vi "TWM Client Cmd Set Measurement.vi"(7 "end of packet key":string="TWM:command:EndOfPacket", 8 "error in":errorcluster, 9 "processing":T1, 10 "meas":T2, 11 "handle":i32) -> (0 "error out":errorcluster, 3 "handle out":i32)   [LabVIEW 2013, in "TWM Client.lvlib"]
doc: "Write Set measurement command packet to TWM server. Sets measurement configuration and processing configuration. The item \"valid?\" of the cluster(s) must be set to \"True\" to send the setup."
uses:
  TWM Client.lvlib
  TWM Client Meas Setup.ctl
  TWM Client Processing Setup.ctl
  octave/infolib.lvlibp/Private/Add key polymorph parts/EXT.vi
  octave/infolib.lvlibp/Private/Add key polymorph parts/I64.vi
  octave/infolib.lvlibp/Private/Add matrix polymorph parts/1D EXT.vi
  octave/infolib.lvlibp/Private/Add key polymorph parts/String.vi
  octave/infolib.lvlibp/Private/Add matrix polymorph parts/1D String.vi
  octave/infolib.lvlibp
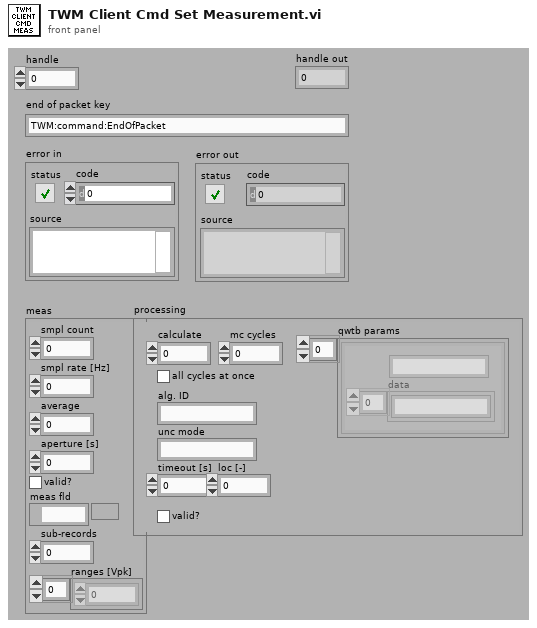
[diagram p1: front panel]
types:
  T1 = typedef "TWM Client.lvlib/TWM Client Processing Setup.ctl" = cluster{"calculate":i32, "all cycles at once":bool, "alg. ID":string, "unc mode":string, "mc cycles":i32, "timeout [s]":dbl, "loc [-]":dbl, "valid?":bool, "qwtb params":cluster{"name":string, "data":string[]}[]}
  T2 = typedef "TWM Client.lvlib/TWM Client Meas Setup.ctl" = cluster{"smpl count":i32, "smpl rate [Hz]":dbl, "average":i32, "aperture [s]":dbl, "valid?":bool, "meas fld":path, "sub-records":i32, "ranges [Vpk]":dbl[]}
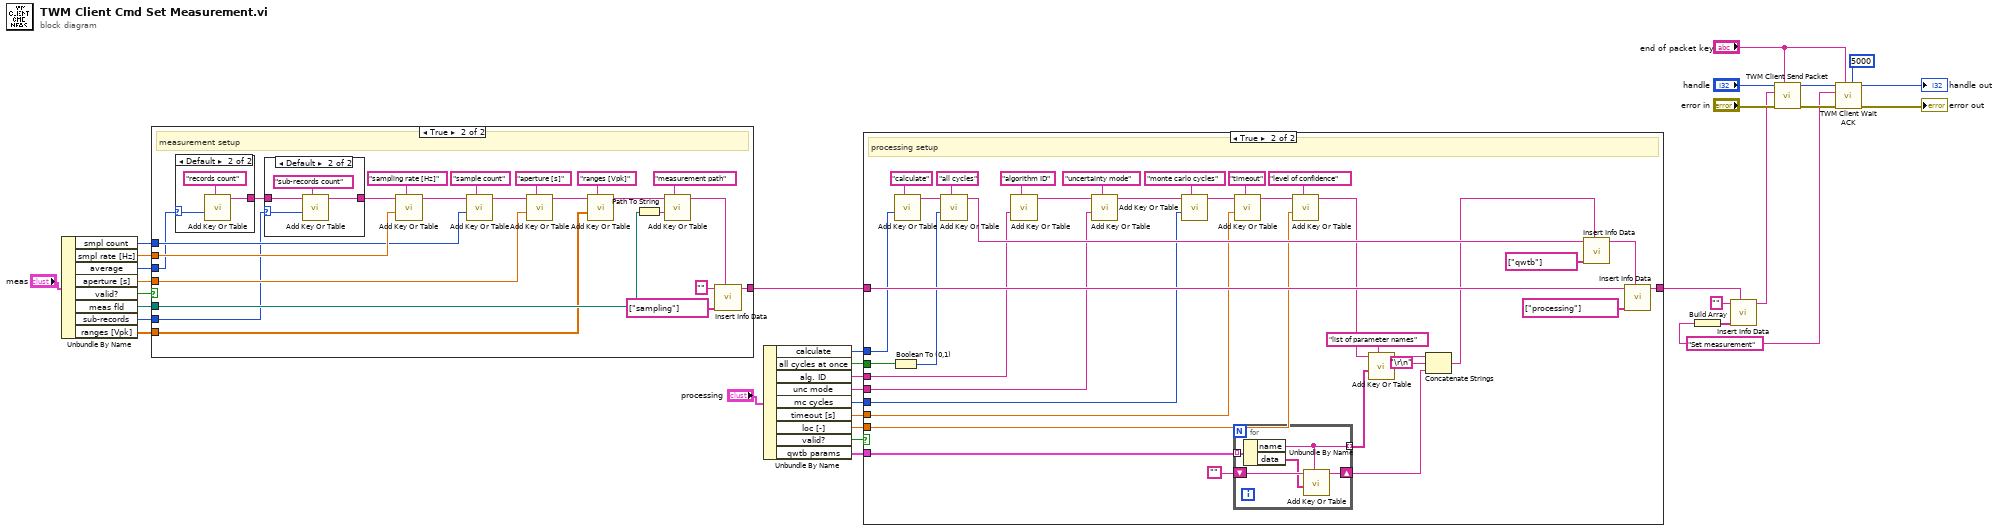
[diagram p0: block diagram]
diagram:
  w3 = "Set measurement" ("section name")
  n1 = Unbundle By Name("meas") -> ("smpl count"=w27:i32, "smpl rate [Hz]"=w28:dbl, "average"=w29:i32, "aperture [s]"=w26:dbl, "valid?"=w25:bool, "meas fld"=w10:path, "sub-records"=w2:i32, "ranges [Vpk]"=w1:dbl[])
  n2 = case shown="True" w25 {
    tunnel: [_ w56] -> w31
    tunnel: w29 -> [_ w39]
    tunnel: w28 -> [_ w51]
    tunnel: w27 -> [_ w50]
    tunnel: w26 -> [_ w49]
    tunnel: w10 -> [_ w44]
    tunnel: w2 -> [_ w40]
    tunnel: w1 -> [_ w34]
    frame False {
    }
    frame True {
      # "measurement setup"
      n3 = case shown="Default" w39 {
        selector: w39 -> [_ w57]
        tunnel: [_ w58] -> w42
        frame 0 {
        }
        frame Default {
          n4 = call-poly "Add Key Or Table.vi"("key description"="records count", "numeric"=w57) -> ("info data out"=w58:string)  [unwired: 8 in, 1 out]
        }
      }
      n5 = case shown="Default" w40 {
        selector: w40 -> [_ w61]
        tunnel: w42 -> [w60 w63]
        tunnel: [w60 w62] -> w41
        frame 0 {
        }
        frame Default {
          n6 = call-poly "Add Key Or Table.vi"("key description"="sub-records count", "numeric"=w61, "info data"=w63) -> ("info data out"=w62:string)  [unwired: 7 in, 1 out]
        }
      }
      n7 = call-poly "Add Key Or Table.vi"("key description"="sampling rate [Hz]", "numeric"=w51, "info data"=w41) -> ("info data out"=w53:string)  [unwired: 7 in, 1 out]
      n8 = call-poly "Add Key Or Table.vi"("key description"="sample count", "numeric"=w50, "info data"=w53) -> ("info data out"=w52:string)  [unwired: 7 in, 1 out]
      n9 = call-poly "Add Key Or Table.vi"("key description"="aperture [s]", "numeric"=w49, "info data"=w52) -> ("info data out"=w36:string)  [unwired: 7 in, 1 out]
      n10 = call-poly "Add Key Or Table.vi"("key description"="ranges [Vpk]", "numeric"=w34, "info data"=w36) -> ("info data out"=w35:string)  [unwired: 7 in, 1 out]
      n11 = Path To String(path=w44) -> (string=w43:string)
      n12 = call-poly "Add Key Or Table.vi"("key description"="measurement path", "string"=w43, "info data"=w35) -> ("info data out"=w45:string)  [unwired: 7 in, 1 out]
      n13 = call "Insert Info Data.vi"("info data to insert"=w45, "sections"=string[] ["sampling"], "info data"="") -> ("info data out"=w56:string)  [unwired: 7 in, 1 out]
    }
  }
  n14 = Unbundle By Name("processing") -> ("calculate"=w23:i32, "all cycles at once"=w22:bool, "alg. ID"=w21:string, "unc mode"=w20:string, "mc cycles"=w19:i32, "timeout [s]"=w18:dbl, "loc [-]"=w17:dbl, "valid?"=w16:bool, "qwtb params"=w11:cluster{"name":string, "data":string[]}[])
  n15 = case shown="True" w16 {
    tunnel: w31 -> [w65 w100]
    tunnel: w23 -> [_ w83]
    tunnel: w22 -> [_ w82]
    tunnel: w21 -> [_ w80]
    tunnel: w20 -> [_ w79]
    tunnel: w19 -> [_ w78]
    tunnel: w18 -> [_ w77]
    tunnel: w17 -> [_ w76]
    tunnel: [w65 w75] -> w15
    tunnel: w11 -> [_ w73]
    frame False {
    }
    frame True {
      # "processing setup"
      n16 = Boolean To (0,1)(Boolean=w82) -> (0, 1=w81:i16)
      n17 = call-poly "Add Key Or Table.vi"("key description"="calculate", "numeric"=w83) -> ("info data out"=w97:string)  [unwired: 8 in, 1 out]
      n18 = call-poly "Add Key Or Table.vi"("key description"="all cycles", "numeric"=w81, "info data"=w97) -> ("info data out"=w84:string)  [unwired: 7 in, 1 out]
      n19 = call-poly "Add Key Or Table.vi"("key description"="algorithm ID", "string"=w80) -> ("info data out"=w98:string)  [unwired: 8 in, 1 out]
      n20 = call-poly "Add Key Or Table.vi"("key description"="uncertainty mode", "string"=w79, "info data"=w98) -> ("info data out"=w88:string)  [unwired: 7 in, 1 out]
      n21 = call-poly "Add Key Or Table.vi"("key description"="monte carlo cycles", "numeric"=w78, "info data"=w88) -> ("info data out"=w90:string)  [unwired: 7 in, 1 out]
      n22 = for {
        tunnel: w73 -> [w105] mode=indexing
        tunnel: [w104] -> w67 mode=indexing
        shift-right: [w102] -> w66
        shift-left: "" -> [w103]
        n23 = Unbundle By Name(w105) -> ("name"=w104:string, "data"=w101:string[])
        n24 = call-poly "Add Key Or Table.vi"("key description"=w104, "string"=w101, "info data"=w103) -> ("info data out"=w102:string)  [unwired: 7 in, 1 out]
      }
      n25 = call-poly "Add Key Or Table.vi"("key description"="timeout", "numeric"=w77, "info data"=w90) -> ("info data out"=w87:string)  [unwired: 7 in, 1 out]
      n26 = call-poly "Add Key Or Table.vi"("key description"="level of confidence", "numeric"=w76, "info data"=w87) -> ("info data out"=w69:string)  [unwired: 7 in, 1 out]
      n27 = call-poly "Add Key Or Table.vi"("key description"="list of parameter names", "string"=w67, "info data"=w69) -> ("info data out"=w71:string)  [unwired: 7 in, 1 out]
      n28 = Concatenate Strings(w71, "\r\n", w66) -> (w68:string)
      n29 = call "Insert Info Data.vi"("info data to insert"=w68, "sections"=string[] ["qwtb"], "info data"=w84) -> ("info data out"=w85:string)  [unwired: 7 in, 1 out]
      n30 = call "Insert Info Data.vi"("info data to insert"=w85, "sections"=string[] ["processing"], "info data"=w100) -> ("info data out"=w75:string)  [unwired: 7 in, 1 out]
    }
  }
  n31 = Build Array(w3) -> (w13:string[])
  n32 = call "Insert Info Data.vi"("info data to insert"=w15, "sections"=w13, "info data"="") -> ("info data out"=w14:string)  [unwired: 7 in, 1 out]
  n33 = call "TWM Client Send Packet.vi"("end of packet key"="end of packet key", "error in"="error in", "command string"=w14, "handle"="handle") -> ("error out"=w9:errorcluster, "handle out"=w8:i32)  [unwired: 6 in]
  n34 = call "TWM Client Wait ACK.vi"("timeout [ms] (3000)"=5000 ("timeout [ms] (1000)"), "key string"="end of packet key", "error in"=w9, "command header"=w3, "handle"=w8) -> ("error out"=→"error out":errorcluster, "handle out"=→"handle out":i32)  [unwired: 5 in]
